vi "_folderExistOrNot_UpData-demo_vna_wmg.vi"(1 "基础路径":path) -> (0 "output":string[](array[string]))   [LabVIEW 2011]
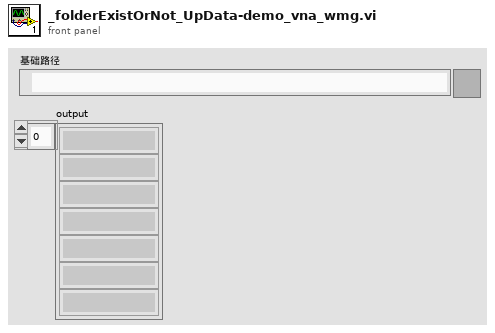
[diagram p1: front panel]
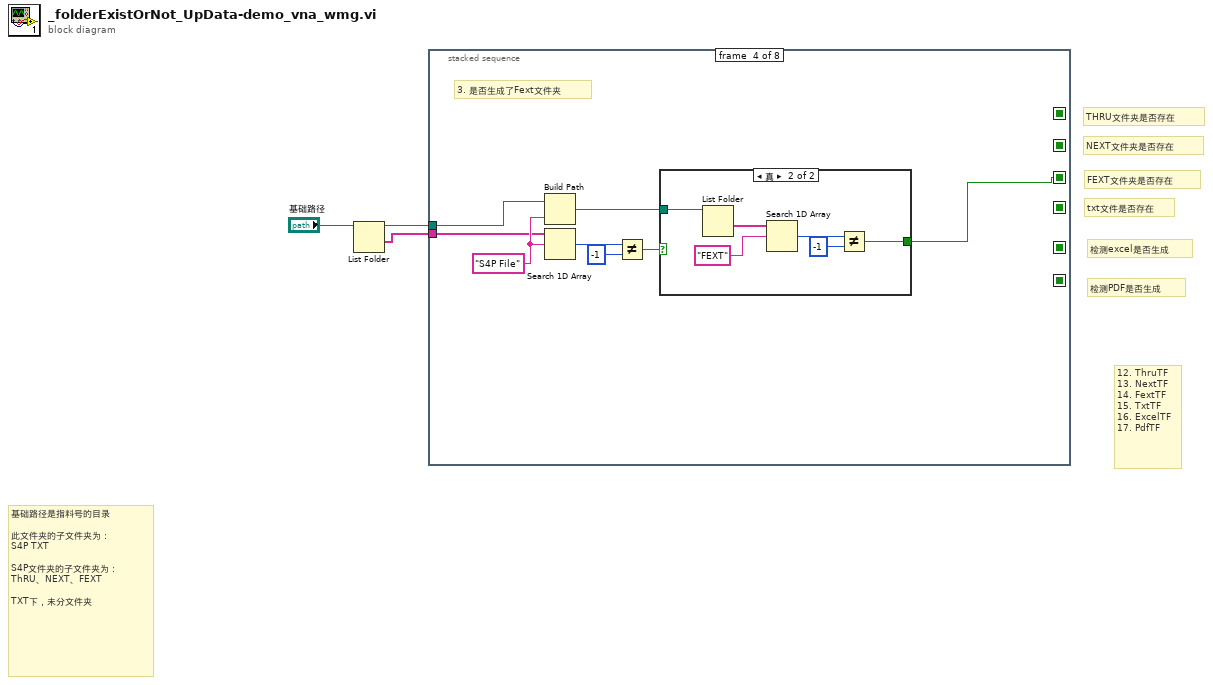
[diagram p0: block diagram]
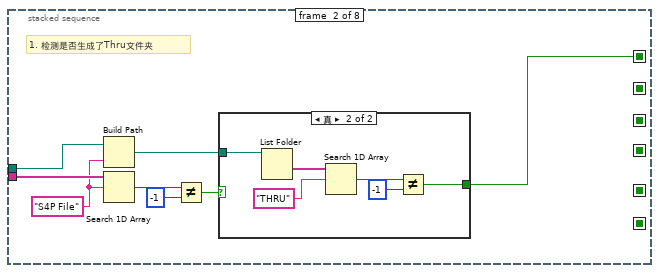
[diagram p3: hidden frame]
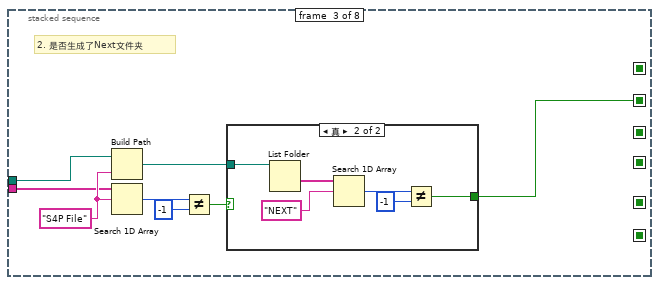
[diagram p5: hidden frame]
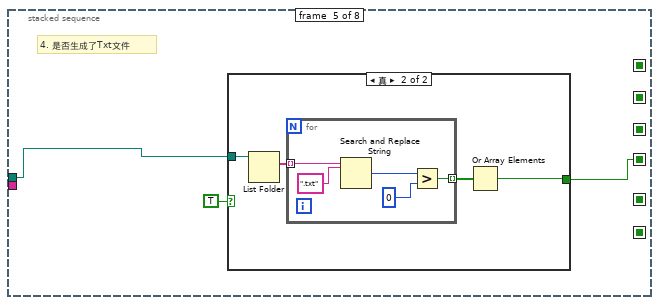
[diagram p8: hidden frame]
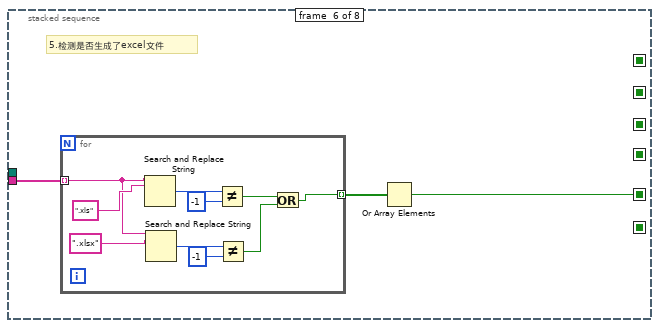
[diagram p10: hidden frame]
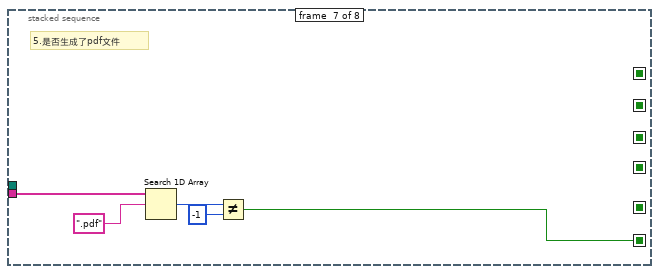
[diagram p11: hidden frame]
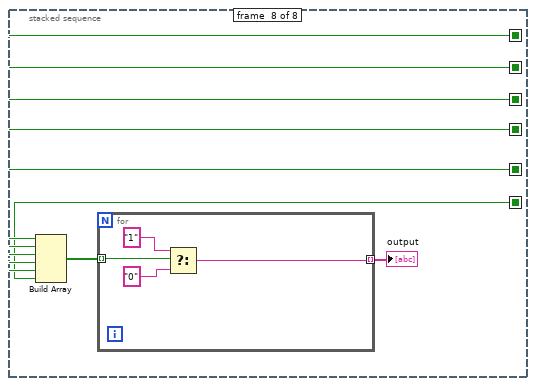
[diagram p12: hidden frame]
diagram:
  # "检测PDF是否生成"
  # "检测excel是否生成"
  # "12. ThruTF\n13. NextTF\n14. FextTF\n15. TxtTF\n16. ExcelTF\n17. PdfTF"
  # "THRU文件夹是否存在"
  # "NEXT文件夹是否存在"
  # "FEXT文件夹是否存在"
  # "txt文件是否存在"
  # "基础路径是指料号的目录\n\n此文件夹的子文件夹为：\nS4P TXT\n\nS4P文件夹的子文件夹为：\nThRU、NEXT、FEXT\n\nTXT下，未分文件夹"
  n1 = List Folder(path="基础路径") -> (path out=w2:path, folder names=w1:string[])  [unwired: 3 in, 2 out]
  n2 = stacked-sequence {
    seq-local: [_ _ _ _ w51 _ _ _] -> [_ _ _ _ _ _ _ w84]
    seq-local: [_ _ _ w34 _ _ _ _] -> [_ _ _ _ _ _ _ w85]
    seq-local: [_ _ w19 _ _ _ _ _] -> [_ _ _ _ _ _ _ w86]
    seq-local: [_ w4 _ _ _ _ _ _] -> [_ _ _ _ _ _ _ w87]
    seq-local: [_ _ _ _ _ w62 _ _] -> [_ _ _ _ _ _ _ w83]
    seq-local: [_ _ _ _ _ _ w75 _] -> [_ _ _ _ _ _ _ w82]
    tunnel: w1 -> [_ w11 w20 w35 _ w64 w76 _]
    tunnel: w2 -> [_ w7 w21 w36 w50 _ _ _]
    frame #0 {
    }
    frame #1 {
      w6 = "S4P File"
      # "1. 检测是否生成了Thru文件夹"
      n3 = Build Path(base path=w7, name or relative path=w6) -> (appended path=w5:path)
      n4 = Search 1D Array(1D array=w11, element=w6) -> (index of element=w10:i32)  [unwired: 1 in]
      n5 = Not Equal?(x=w10, y=-1) -> (x != y?=w8:bool)
      n6 = case shown="真" w8 {
        selector: w8 -> [w12 _]
        tunnel: w5 -> [_ w15]
        tunnel: [w12 w13] -> w4
        frame False {
        }
        frame True {
          n7 = List Folder(path=w15) -> (folder names=w14:string[])  [unwired: 3 in, 3 out]
          n8 = Search 1D Array(1D array=w14, element="THRU") -> (index of element=w17:i32)  [unwired: 1 in]
          n9 = Not Equal?(x=w17, y=-1) -> (x != y?=w13:bool)
        }
      }
    }
    frame #2 {
      w23 = "S4P File"
      # "2. 是否生成了Next文件夹"
      n10 = Build Path(base path=w21, name or relative path=w23) -> (appended path=w22:path)
      n11 = Search 1D Array(1D array=w20, element=w23) -> (index of element=w26:i32)  [unwired: 1 in]
      n12 = Not Equal?(x=w26, y=-1) -> (x != y?=w24:bool)
      n13 = case shown="真" w24 {
        selector: w24 -> [w27 _]
        tunnel: w22 -> [_ w30]
        tunnel: [w27 w28] -> w19
        frame False {
        }
        frame True {
          n14 = List Folder(path=w30) -> (folder names=w29:string[])  [unwired: 3 in, 3 out]
          n15 = Search 1D Array(1D array=w29, element="NEXT") -> (index of element=w32:i32)  [unwired: 1 in]
          n16 = Not Equal?(x=w32, y=-1) -> (x != y?=w28:bool)
        }
      }
    }
    frame #3 {
      w38 = "S4P File"
      # "3. 是否生成了Fext文件夹"
      n17 = Build Path(base path=w36, name or relative path=w38) -> (appended path=w37:path)
      n18 = Search 1D Array(1D array=w35, element=w38) -> (index of element=w41:i32)  [unwired: 1 in]
      n19 = Not Equal?(x=w41, y=-1) -> (x != y?=w39:bool)
      n20 = case shown="真" w39 {
        selector: w39 -> [w42 _]
        tunnel: w37 -> [_ w45]
        tunnel: [w42 w43] -> w34
        frame False {
        }
        frame True {
          n21 = List Folder(path=w45) -> (folder names=w44:string[])  [unwired: 3 in, 3 out]
          n22 = Search 1D Array(1D array=w44, element="FEXT") -> (index of element=w47:i32)  [unwired: 1 in]
          n23 = Not Equal?(x=w47, y=-1) -> (x != y?=w43:bool)
        }
      }
    }
    frame #4 {
      # "4. 是否生成了Txt文件"
      n24 = case shown="真" TRUE {
        selector: TRUE -> [w52 _]
        tunnel: w50 -> [_ w56]
        tunnel: [w52 w53] -> w51
        frame False {
        }
        frame True {
          n25 = List Folder(path=w56) -> (filenames=w54:string[])  [unwired: 3 in, 3 out]
          n26 = for {
            tunnel: [w59] -> w55 mode=indexing
            tunnel: w54 -> [w58] mode=indexing
            n27 = Search and Replace String(input string=w58, search string=".txt" ("元素")) -> (number of replacements=w60:i32)  [unwired: 6 in, 3 out]
            n28 = Greater?(x=w60, y=0) -> (0:w59:bool)
          }
          n29 = Or Array Elements(Boolean array=w55) -> (logical OR=w53:bool)
        }
      }
    }
    frame #5 {
      # "5.检测是否生成了excel文件"
      n30 = for {
        tunnel: w64 -> [w66] mode=indexing
        tunnel: [w68] -> w63 mode=indexing
        n31 = Search and Replace String(input string=w66, search string=".xls") -> (number of replacements=w74:i32)  [unwired: 6 in, 3 out]
        n32 = Search and Replace String(input string=w66, search string=".xlsx") -> (number of replacements=w71:i32)  [unwired: 6 in, 3 out]
        n33 = Not Equal?(x=w74, y=-1) -> (x != y?=w70:bool)
        n34 = Not Equal?(x=w71, y=-1) -> (x != y?=w69:bool)
        n35 = Or(x=w70, y=w69) -> (x .or. y?=w68:bool)
      }
      n36 = Or Array Elements(Boolean array=w63) -> (logical OR=w62:bool)
    }
    frame #6 {
      # "5.是否生成了pdf文件"
      n37 = Search 1D Array(1D array=w76, element=".pdf") -> (index of element=w79:i32)  [unwired: 1 in]
      n38 = Not Equal?(x=w79, y=-1) -> (x != y?=w75:bool)
    }
    frame #7 {
      n39 = Build Array(w87, w86, w85, w84, w83, w82) -> (w81:bool[])
      n40 = for {
        tunnel: w81 -> [w91] mode=indexing
        tunnel: [w88] -> w80 mode=indexing
        n41 = Select(t="1", s=w91, f="0") -> (s? t:f=w88:string)
      }
      "output" <- w80
    }
  }
